vi "Clear Hardware.vi"(2 "error in (no error)":errorcluster, 3 "SRS_SG380 in":refnum<class "SRS_SG380.lvclass">) -> (0 "error out":errorcluster, 1 "SRS_SG380 out":refnum<class "SRS_SG380.lvclass">)   [LabVIEW 2013, in "SRS_SG380.lvclass"]
doc: "This VI resets any necessary hardware so that the device will be ready for the next run."
uses:
  SRS_SG380.lvclass
  Device/Device.lvclass
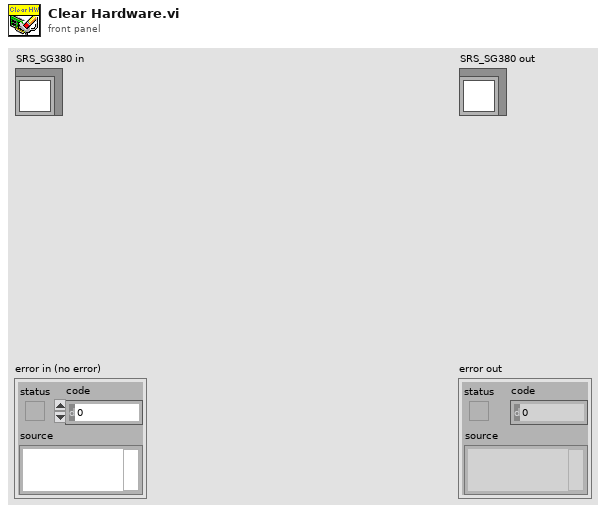
[diagram p1: front panel]
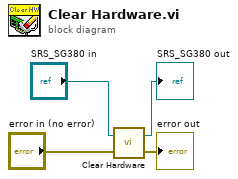
[diagram p0: block diagram]
diagram:
  n1 = call-parent "Clear Hardware.vi"("error in (no error)"="error in (no error)", "Device in"="SRS_SG380 in") -> ("error out"=→"error out":errorcluster, "Device out"=→"SRS_SG380 out":refnum<class "SRS_SG380.lvclass">)
